vi "ReadConnectionReference.vi"(8 "error in (no error)":errorcluster, 11 "object in":refnum<class "Database.lvclass">) -> (0 "error out":errorcluster, 2 "connection reference":T1, 3 "object out":refnum<class "Database.lvclass">)   [LabVIEW 2023, in "HardwareAbstractionLayer_LVOOP.lvlib" / "Database.lvclass"]
doc: "Get Conncetion Reference"
uses:
  Database.lvclass
  <vilib>/addons/database/Connection.llb/Conn ObjectReference.ctl
  Database.lvclass/Database.ctl
  <vilib>/addons/database/NI_Database_API.lvlib
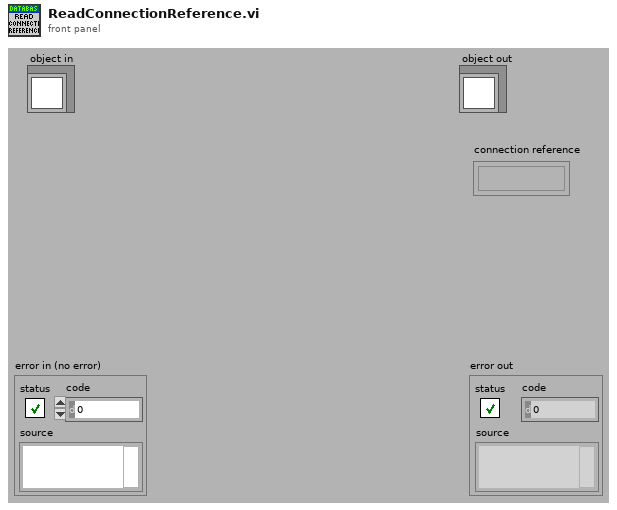
[diagram p1: front panel]
types:
  T1 = typedef "NI_Database_API.lvlib/Conn ObjectReference.ctl" = refnum<k1>
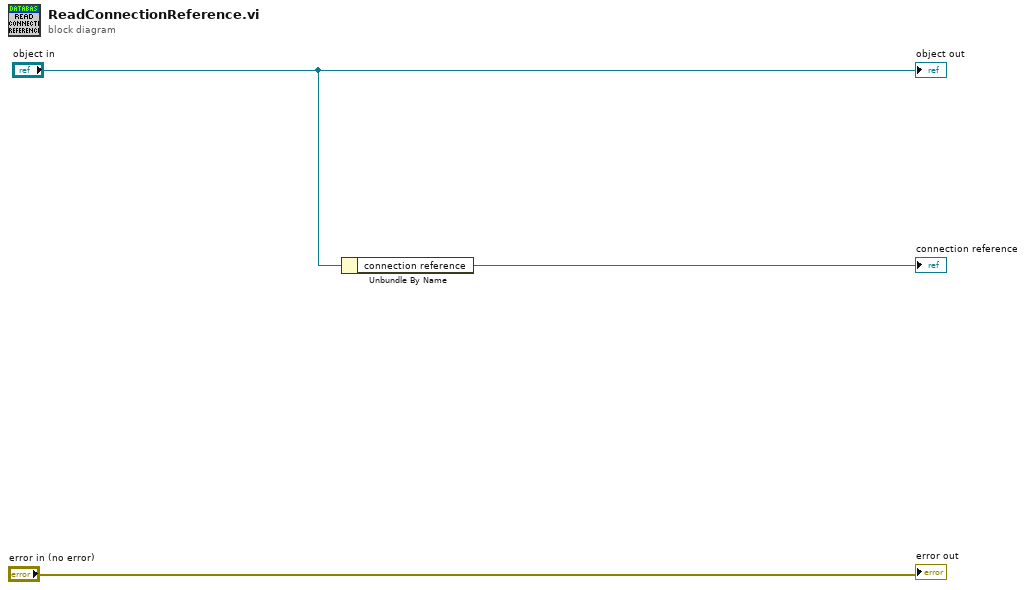
[diagram p0: block diagram]
diagram:
  n1 = Unbundle By Name("object in") -> ("connection reference"=→"connection reference":T1)
  "error out" <- "error in (no error)"
  "object out" <- "object in"
